vi "Gif.ImageDescriptor.vi"(0 "data":string, 9 "offset":i32, 11 "error in (no error)":errorcluster) -> (4 "data out":string, 10 "offset out":i32, 14 "ImageDescriptor":T1, 15 "error out":errorcluster)   [LabVIEW 2011]
uses:
  Gif.ImageDescriptor.ctl
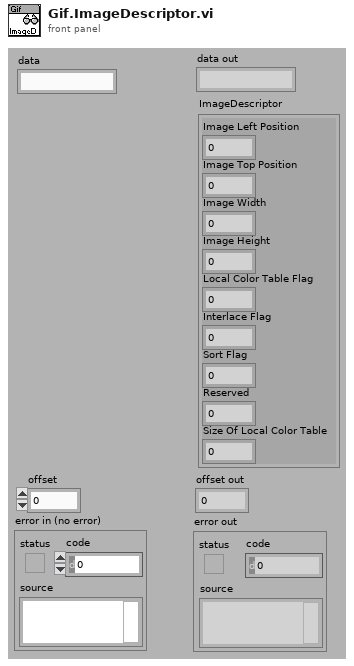
[diagram p1: front panel]
types:
  T1 = typedef "Gif.ImageDescriptor.ctl" = cluster{"Image Left Position":u16, "Image Top Position":u16, "Image Width":u16, "Image Height":u16, "Local Color Table Flag":u8, "Interlace Flag":u8, "Sort Flag":u8, "Reserved":u8, "Size Of Local Color Table":u8}
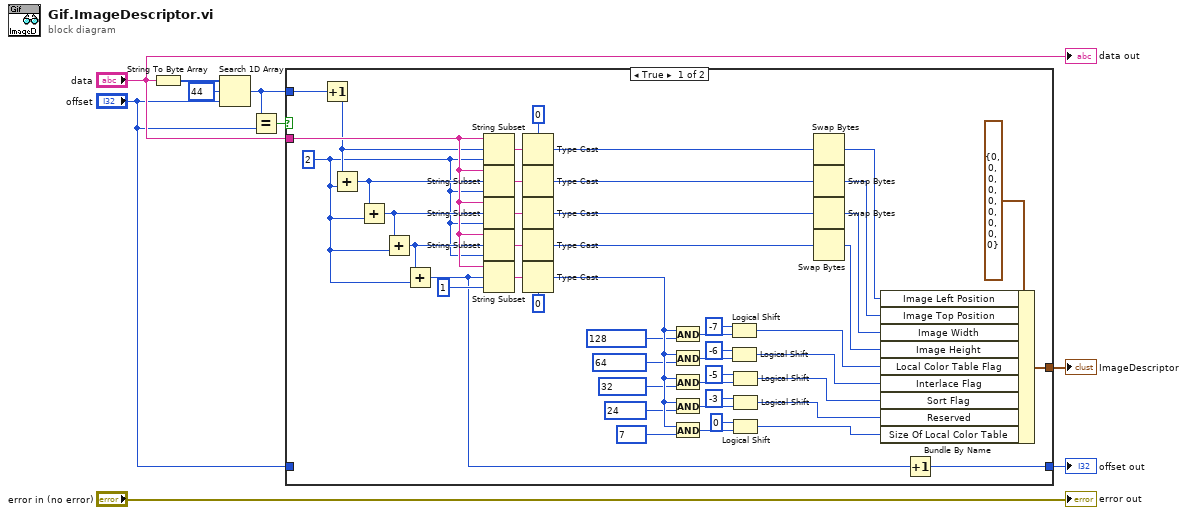
[diagram p0: block diagram]
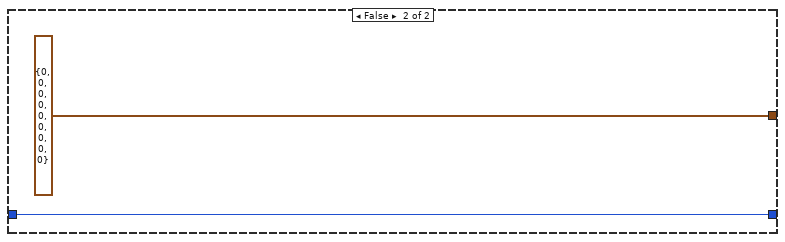
[diagram p2: hidden frame]
diagram:
  n1 = String To Byte Array(string="data") -> (unsigned byte array=w9:u8[])
  n2 = Search 1D Array(1D array=w9, element=u8 44, start index (0)="offset") -> (index of element=w2:i32)
  n3 = Equal?(x=w2, y="offset") -> (x = y?=w3:bool)
  n4 = case shown="True" w3 {
    tunnel: "data" -> [w57 _]
    tunnel: [w27 T1 {"Image Left Position"=0, "Image Top Position"=0, "Image Width"=0, "Image Height"=0, "Local Color Table Flag"=0, "Interlace Flag"=0, "Sort Flag"=0, "Reserved"=0, "Size Of Local Color Table"=0} ("ImageDescriptor")] -> w6
    tunnel: [w26 w59] -> w5
    tunnel: "offset" -> [_ w59]
    tunnel: w2 -> [w25 _]
    frame True {
      w45 = u16 0 ("length (rest)")
      w52 = 2 ("length (rest)")
      n5 = Increment(x=w25) -> (x+1=w56:i32)
      n6 = Add(x=w56, y=w52) -> (x+y=w55:i32)
      n7 = Add(x=w55, y=w52) -> (x+y=w54:i32)
      n8 = Add(x=w54, y=w52) -> (x+y=w53:i32)
      n9 = Add(x=w53, y=w52) -> (x+y=w50:i32)
      n10 = String Subset(string=w57, offset (0)=w56, length (rest)=w52) -> (substring=w49:string)
      n11 = String Subset(string=w57, offset (0)=w55, length (rest)=w52) -> (substring=w48:string)
      n12 = String Subset(string=w57, offset (0)=w54, length (rest)=w52) -> (substring=w47:string)
      n13 = String Subset(string=w57, offset (0)=w53, length (rest)=w52) -> (substring=w46:string)
      n14 = String Subset(string=w57, offset (0)=w50, length (rest)=1 ("length (rest)")) -> (substring=w40:string)
      n15 = Type Cast(type=w45, x=w49) -> (*(type *) &x=w44:u16)
      n16 = Type Cast(type=w45, x=w48) -> (*(type *) &x=w43:u16)
      n17 = Type Cast(type=w45, x=w47) -> (*(type *) &x=w42:u16)
      n18 = Type Cast(type=w45, x=w46) -> (*(type *) &x=w41:u16)
      n19 = Type Cast(type=u8 0 ("length (rest)"), x=w40) -> (*(type *) &x=w38:u8)
      n20 = And(x=w38, y=u8 128 ("length (rest)")) -> (x .and. y?=w19:u8)
      n21 = And(x=w38, y=u8 64 ("length (rest)")) -> (x .and. y?=w18:u8)
      n22 = And(x=w38, y=u8 32 ("length (rest)")) -> (x .and. y?=w17:u8)
      n23 = And(x=w38, y=u8 24 ("length (rest)")) -> (x .and. y?=w16:u8)
      n24 = And(x=w38, y=u8 7 ("length (rest)")) -> (x .and. y?=w15:u8)
      n25 = Logical Shift(y=-7 ("length (rest)"), x=w19) -> (x << y=w32:u8)
      n26 = Logical Shift(y=-6 ("length (rest)"), x=w18) -> (x << y=w33:u8)
      n27 = Logical Shift(y=-5 ("length (rest)"), x=w17) -> (x << y=w34:u8)
      n28 = Logical Shift(y=-3 ("length (rest)"), x=w16) -> (x << y=w35:u8)
      n29 = Logical Shift(y=0 ("length (rest)"), x=w15) -> (x << y=w36:u8)
      n30 = Swap Bytes(anything=w44) -> (byte swapped=w31:u16)
      n31 = Swap Bytes(anything=w43) -> (byte swapped=w28:u16)
      n32 = Swap Bytes(anything=w42) -> (byte swapped=w29:u16)
      n33 = Swap Bytes(anything=w41) -> (byte swapped=w30:u16)
      n34 = Bundle By Name(cluster=T1 {"Image Left Position"=0, "Image Top Position"=0, "Image Width"=0, "Image Height"=0, "Local Color Table Flag"=0, "Interlace Flag"=0, "Sort Flag"=0, "Reserved"=0, "Size Of Local Color Table"=0} ("ImageDescriptor"), "Image Left Position"=w31, "Image Top Position"=w28, "Image Width"=w29, "Image Height"=w30, "Local Color Table Flag"=w32, "Interlace Flag"=w33, "Sort Flag"=w34, "Reserved"=w35, "Size Of Local Color Table"=w36) -> (w27:T1)
      n35 = Increment(x=w50) -> (x+1=w26:i32)
    }
    frame False {
    }
  }
  "ImageDescriptor" <- w6
  "offset out" <- w5
  "data out" <- "data"
  "error out" <- "error in (no error)"
